vi "Get Application Instances.vi"(8 "error in (no error)":errorcluster, 11 "Update":bool) -> (0 "error out":errorcluster, 1 "Valid":bool, 2 "App Instance Names":string[](array[string]), 3 "App Instances":refnum<vi>[](array[refnum]))   [LabVIEW 2013, in "LVTM.lvlib"]
uses:
  LVTM.lvlib
  <vilib>/Utility/error.llb/DialogType.ctl
panel:
  in  "Cancel":bool
  in  "Machine name":string="localhost"
  in  "Port number":u16=3363
  # "Select Application Instance"
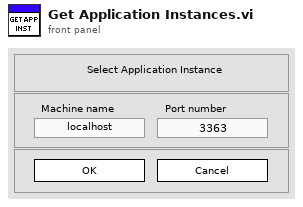
[diagram p1: front panel]
types:
  T1 = enum32{"Invalid", "Standard", "Closed", "Hidden", "Minimized", "Maximized"}
  T2 = typedef "DialogType.ctl" = u16
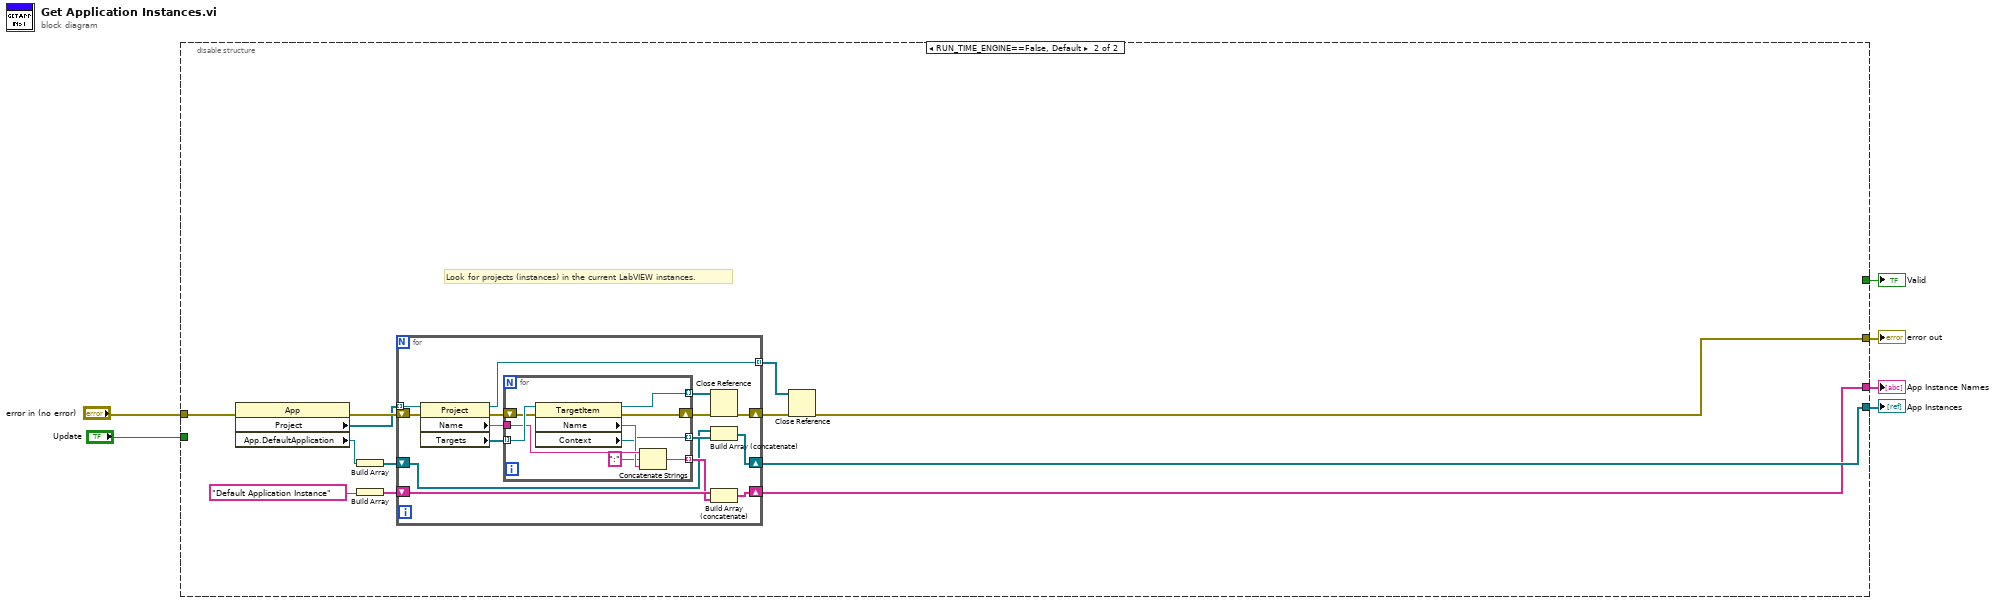
[diagram p0: block diagram]
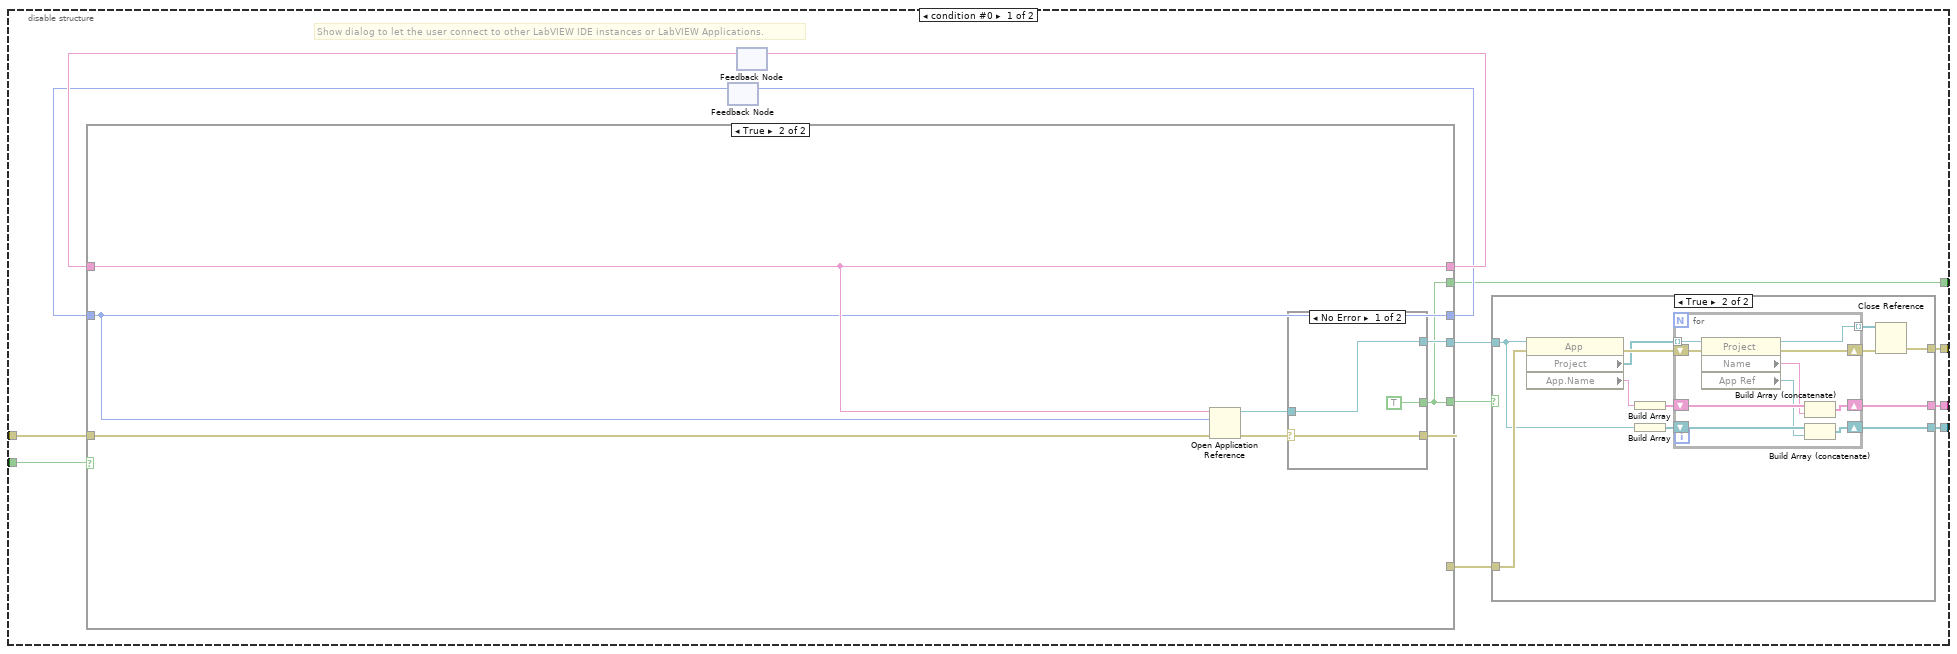
[diagram p2: hidden frame]
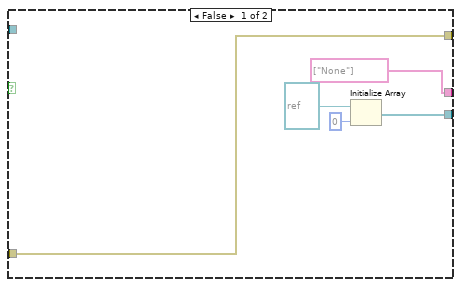
[diagram p3: hidden frame]
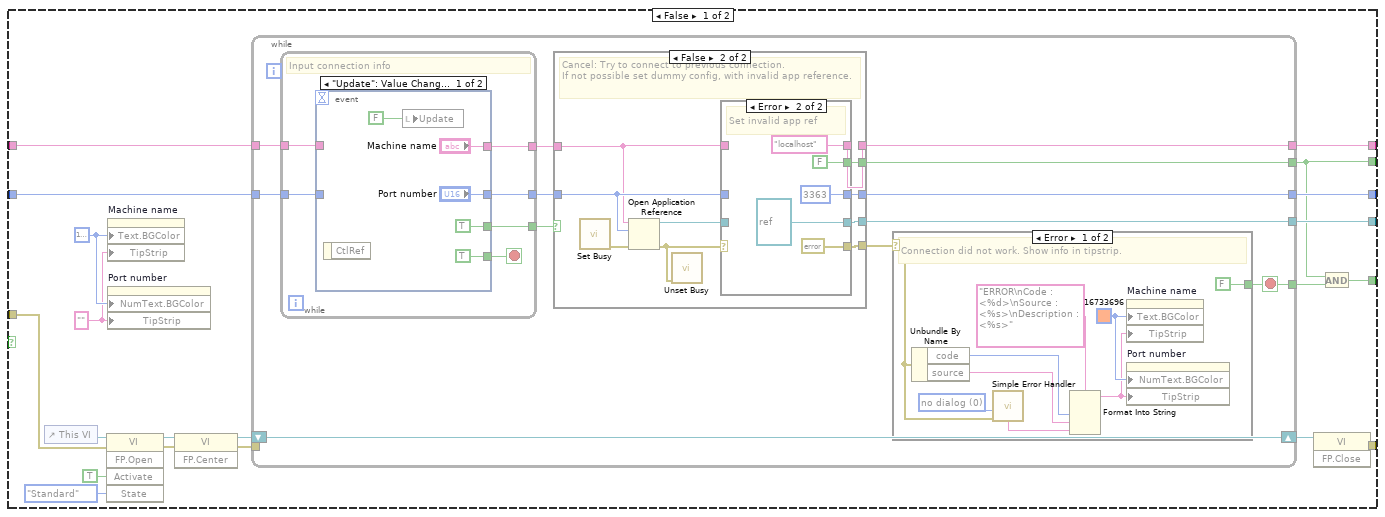
[diagram p4: hidden frame]
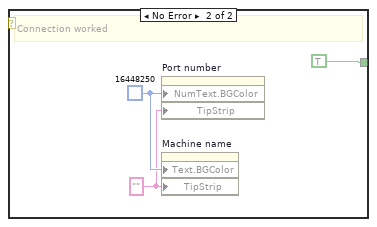
[diagram p5: hidden frame]
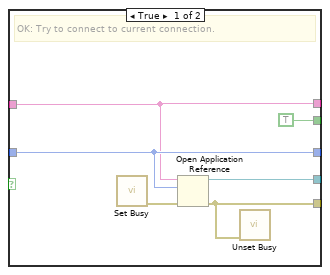
[diagram p6: hidden frame]
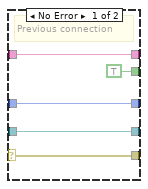
[diagram p7: hidden frame]
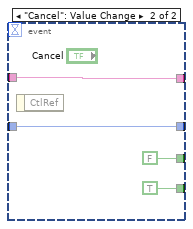
[diagram p8: hidden frame]
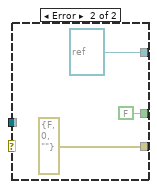
[diagram p9: hidden frame]
diagram:
  n1 = disable-structure shown="RUN_TIME_ENGINE==False, Default" {
    disable-tunnel: [w19 w148] -> w6
    disable-tunnel: "Update" -> [w18 _]
    disable-tunnel: "error in (no error)" -> [w17 w149]
    disable-tunnel: [w10 w147] -> w3
    disable-tunnel: [w9 w146] -> w2
    disable-tunnel: [w7 _] -> w1
    frame condition #0 {
      # "Show dialog to let the user connect to other LabVIEW IDE instances or LabVIEW Applications."
      n2 = feedback #1() -> (w11:u16)  [unwired: 1 in]
      n3 = feedback #2() -> (w13:string)  [unwired: 1 in]
      n4 = case shown="True" w18 {
        tunnel: w17 -> [w50 w139]
        tunnel: [w60 w133] -> w15
        tunnel: [w59 w135] -> w16
        tunnel: [w54 w138] -> w14
        tunnel: [w53 w137] -> w12
        tunnel: w13 -> [w55 w138]
        tunnel: w11 -> [w56 w137]
        tunnel: [w51 w132] -> w8
        tunnel: [w47 w132] -> w7
        frame False {
          w57 = "" ("Tip Strip")
          w58 = u32 16777226
          n5 = control-ref of="This VI"() -> (w66:refnum<vi>)
          n6 = invoke class="VI" method="FP.Open"(reference=w66, error in=w50, "Activate"=TRUE ("Activate?"), "State"=T1."Standard") -> (reference out=w62:refnum<vi>, error out=w49:errorcluster)  [unwired: 1 in, 3 out]
          n7 = property on="Machine name" class="Str"("Text.BGColor"=w58, "TipStrip"=w57) -> ()  [unwired: 2 in, 2 out]
          n8 = property on="Port number" class="DigNum (strict)"("NumText.BGColor"=w58, "TipStrip"=w57) -> ()  [unwired: 2 in, 2 out]
          n9 = invoke class="VI" method="FP.Center"(reference=w62, error in=w49) -> (reference out=w61:refnum<vi>, error out=w48:errorcluster)  [unwired: 1 in, 1 out]
          n10 = while {
            tunnel: w55 -> [w70]
            tunnel: w56 -> [w69]
            shift-right: [w78] -> w63
            shift-left: w61 -> [w78]
            tunnel: [w77] -> w60
            tunnel: [w68] -> w54
            tunnel: [w67] -> w53
            tunnel: [w73] -> w52
            tunnel: [w71] -> w47
            tunnel: w48 -> [_]
            stop <- w73 stop-if-true
            n11 = while {
              tunnel: [w122] -> w76
              tunnel: [w121] -> w75
              tunnel: w70 -> [w119]
              tunnel: w69 -> [w118]
              tunnel: [w117] -> w72
              stop <- w120 stop-if-true
              # "Input connection info"
              n12 = event shown="[0] \"Update\": Value Change" {
                selector: _ -> [_ _]
                dyn-events: _ -> [_ _]
                timeout: _ -> [_ _]
                tunnel: ["Port number" w130] -> w122
                tunnel: ["Machine name" w131] -> w121
                tunnel: [TRUE TRUE] -> w120
                tunnel: w119 -> [_ w131]
                tunnel: w118 -> [_ w130]
                tunnel: [TRUE FALSE] -> w117
                event "Update": Value Change {
                  n13 = event-data() -> ()  [unwired: 1 in, 1 out]
                  n14 = local write "Update"(FALSE ("OK Button")) -> ()
                }
                event "Cancel": Value Change {
                  n15 = event-data() -> ()  [unwired: 1 in, 1 out]
                }
              }
            }
            n16 = case shown="False" w72 {
              tunnel: w76 -> [w93 w101]
              tunnel: w75 -> [w92 w99]
              tunnel: [w95 w104] -> w74
              tunnel: [w96 w102] -> w77
              tunnel: [w92 w100] -> w68
              tunnel: [w93 w98] -> w67
              tunnel: [TRUE w97] -> w71
              frame True {
                # "OK: Try to connect to current connection."
                n17 = call <vilib>:"Set Busy.vi"() -> ("error out"=w94:errorcluster)  [unwired: 10 in, 1 out]
                n18 = Open Application Reference(8:w94, 10:w93, 11:w92) -> (0:w95:errorcluster, 3:w96:refnum<vi>)  [unwired: 1 in]
                n19 = call <vilib>:"Unset Busy.vi"("error in (no error)"=w95) -> ()  [unwired: 10 in, 1 out]
              }
              frame False {
                # "Cancel: Try to connect to previous connection.\nIf not possible set dummy config, with invalid app reference."
                n20 = call <vilib>:"Set Busy.vi"() -> ("error out"=w106:errorcluster)  [unwired: 10 in, 1 out]
                n21 = Open Application Reference(8:w106, 10:w101, 11:w99) -> (0:w105:errorcluster, 3:w103:refnum<vi>)  [unwired: 1 in]
                n22 = call <vilib>:"Unset Busy.vi"("error in (no error)"=w105) -> ()  [unwired: 10 in, 1 out]
                n23 = case shown="Error" w105 {
                  selector: w105 -> [w111 _]
                  tunnel: [w111 errorcluster {"status"=FALSE, "code"=0, "source"=""} ("error IO")] -> w104
                  tunnel: w103 -> [w110 _]
                  tunnel: [w110 refnum<vi> refnum ("application reference")] -> w102
                  tunnel: [w108 u16 3363 ("Port number")] -> w98
                  tunnel: w101 -> [w108 _]
                  tunnel: [w109 "localhost" ("Machine name")] -> w100
                  tunnel: w99 -> [w109 _]
                  tunnel: [TRUE FALSE] -> w97
                  frame No Error {
                    # "Previous connection"
                  }
                  frame Error {
                    # "Set invalid app ref"
                  }
                }
              }
            }
            n24 = case shown="Error" w74 {
              selector: w74 -> [w84 _]
              tunnel: [FALSE TRUE] -> w73
              frame Error {
                w85 = T2 0 items=["no dialog", "OK message", "continue or stop message", "OK message + warnings", "continue/stop + warnings"] ("type of dialog (OK msg:1)")
                w87 = u32 16733696
                # "Connection did not work. Show info in tipstrip."
                n25 = Unbundle By Name(w84) -> ("code"=w79:i32, "source"=w82:string)
                n26 = call <vilib>:"Simple Error Handler.vi"("type of dialog (OK msg:1)"=w85, "error in (no error)"=w84) -> ("message"=w83:string)  [unwired: 3 in, 4 out]
                n27 = Format Into String(format string="ERROR\nCode : <%d>\nSource : <%s>\nDescription : <%s>", w79, w82, w83) -> (resulting string=w80:string)  [unwired: 2 in, 1 out]
                n28 = property on="Machine name" class="Str"("Text.BGColor"=w87, "TipStrip"=w80) -> ()  [unwired: 2 in, 2 out]
                n29 = property on="Port number" class="DigNum (strict)"("NumText.BGColor"=w87, "TipStrip"=w80) -> ()  [unwired: 2 in, 2 out]
              }
              frame No Error {
                w88 = "" ("Tip Strip")
                w90 = u32 16448250
                # "Connection worked"
                n30 = property on="Port number" class="DigNum (strict)"("NumText.BGColor"=w90, "TipStrip"=w88) -> ()  [unwired: 2 in, 2 out]
                n31 = property on="Machine name" class="Str"("Text.BGColor"=w90, "TipStrip"=w88) -> ()  [unwired: 2 in, 2 out]
              }
            }
          }
          n32 = invoke class="VI" method="FP.Close"(reference=w63) -> (error out=w59:errorcluster)  [unwired: 2 in, 2 out]
          n33 = And(x=w47, y=w52) -> (x .and. y?=w51:bool)
        }
        frame True {
          n34 = Open Application Reference(8:w139, 10:w137, 11:w138) -> (0:w136:errorcluster, 3:w134:refnum<vi>)  [unwired: 1 in]
          n35 = case shown="No Error" w136 {
            selector: w136 -> [w141 _]
            tunnel: [TRUE FALSE] -> w132
            tunnel: [w141 errorcluster {"status"=FALSE, "code"=0, "source"=""} ("error IO")] -> w135
            tunnel: w134 -> [w140 _]
            tunnel: [w140 refnum<vi> refnum ("application reference")] -> w133
            frame No Error {
            }
            frame Error {
            }
          }
        }
      }
      n36 = feedback-in #1(w12) -> ()
      n37 = feedback-in #2(w14) -> ()
      n38 = case shown="True" w8 {
        tunnel: [w24 w36] -> w19
        tunnel: w15 -> [_ w34]
        tunnel: [w20 w25] -> w10
        tunnel: [string[] ["None"] w26] -> w9
        tunnel: w16 -> [w24 w35]
        frame False {
          n39 = Initialize Array(refnum<vi> refnum ("application reference"), 0 ("dimension size")) -> (w20:refnum<vi>[])
        }
        frame True {
          n40 = property class="App"(reference=w34, error in=w35) -> (error out=w31:errorcluster, "Project"=w30:refnum<vi>[], "App.Name"=w29:string)  [unwired: 1 out]
          n41 = Build Array(w29) -> (w27:string[])
          n42 = Build Array(w34) -> (w28:refnum<vi>[])
          n43 = for {
            tunnel: w30 -> [w43] mode=indexing
            shift-right: [w38] -> w26
            shift-left: w27 -> [w46]
            shift-right: [w41] -> w32
            shift-left: w31 -> [w45]
            shift-right: [w37] -> w25
            shift-left: w28 -> [w44]
            tunnel: [w42] -> w33 mode=indexing
            n44 = property class="Project"(reference=w43, error in=w45) -> (reference out=w42:refnum<vi>, error out=w41:errorcluster, "Name"=w40:string, "App Ref"=w39:refnum<vi>)
            n45 = Build Array (concatenate)(w46, w40) -> (w38:string[])
            n46 = Build Array (concatenate)(w44, w39) -> (w37:refnum<vi>[])
          }
          n47 = Close Reference(reference=w33, error in (no error)=w32) -> (error out=w36:errorcluster)
        }
      }
    }
    frame condition #1 (active) {
      # "Look for projects (instances) in the current LabVIEW instances."
      n48 = property class="App"(error in=w149) -> (error out=w151:errorcluster, "Project"=w150:refnum<vi>[], "App.DefaultApplication"=w156:refnum<vi>)  [unwired: 1 in, 1 out]
      n49 = Build Array(w156) -> (w153:refnum<vi>[])
      n50 = Build Array("Default Application Instance") -> (w152:string[])
      n51 = for {
        tunnel: w150 -> [w162] mode=indexing
        shift-right: [w168] -> w146
        shift-left: w152 -> [w170]
        shift-right: [w160] -> w154
        shift-left: w151 -> [w166]
        shift-right: [w164] -> w147
        shift-left: w153 -> [w163]
        tunnel: [w158] -> w155 mode=indexing
        n52 = property class="Project"(reference=w162, error in=w166) -> (reference out=w158:refnum<vi>, error out=w167:errorcluster, "Name"=w171:string, "Targets"=w172:refnum<vi>[])
        n53 = for {
          tunnel: w172 -> [w181] mode=indexing
          tunnel: w171 -> [w180]
          tunnel: [w177] -> w169 mode=indexing
          shift-right: [w174] -> w161
          shift-left: w167 -> [w176]
          tunnel: [w175] -> w165 mode=indexing
          tunnel: [w173] -> w159 mode=indexing
          n54 = property class="TargetItem"(reference=w181, error in=w176) -> (reference out=w173:refnum<vi>, error out=w174:errorcluster, "Name"=w179:string, "Context"=w175:refnum<vi>)
          n55 = Concatenate Strings(w180, ":" ("string"), w179) -> (w177:string)
        }
        n56 = Close Reference(reference=w159, error in (no error)=w161) -> (error out=w160:errorcluster)
        n57 = Build Array (concatenate)(w163, w165) -> (w164:refnum<vi>[])
        n58 = Build Array (concatenate)(w170, w169) -> (w168:string[])
      }
      n59 = Close Reference(reference=w155, error in (no error)=w154) -> (error out=w148:errorcluster)
    }
  }
  "error out" <- w6
  "App Instance Names" <- w2
  "App Instances" <- w3
  "Valid" <- w1
